vi "Accelerometer Logger.vi"() -> ()   [LabVIEW 2013]
uses:
  Accelerometer Data.ctl
  <vilib>/Platform/TimedLoop/XDataNode/timing_clust.ctl
  <vilib>/Platform/TimedLoop/XDataNode/nitl_modes.ctl
  <vilib>/Platform/TimedLoop/XDataNode/wakeup.ctl
  <vilib>/Analysis/_algsub.llb/Real Vector Norm.vi
  <vilib>/platform/TimedLoop/XDataNode/XDataNode.xnode
  <vilib>/Platform/TimedLoop/XDataNode/XDNodeRunTimeDep.lvlib
  <vilib>/Analysis/NI_AALPro.lvlib
panel:
  in  "ACK timeout":dbl[unit]=0.5
  in  "I2C clock speed":dbl[unit]=100000.0
  in  "reset":bool
  out "file":path caption="File name:"
  in  "increment file":bool
  in  "Stop on trigger":bool=TRUE
  out "error out":errorcluster
  in  "zero":bool
  out "actrate":dbl[unit] caption="Actual rate"
  in  "Post trigger":dbl[unit]=0.5
  out "Trigger":bool
  out "mag":dbl(slide) caption="Magnitude (g)" scale=0.0..2.0
  in  "Stop":bool
  in  "accel range (g)":u16(ring)=2 items=["2"=2, "4"=4, "8"=8, "16"=16]
  in  "gyro range (deg/sec)":u16(ring)=250 items=["250"=250, "500"=500, "1000"=1000, "2000"=2000]
  out "Gyro":waveform(dbl)[](graph)
  out "Accel":waveform(dbl)[](graph)
  in  "Sampling rate":dbl[unit]=200.0
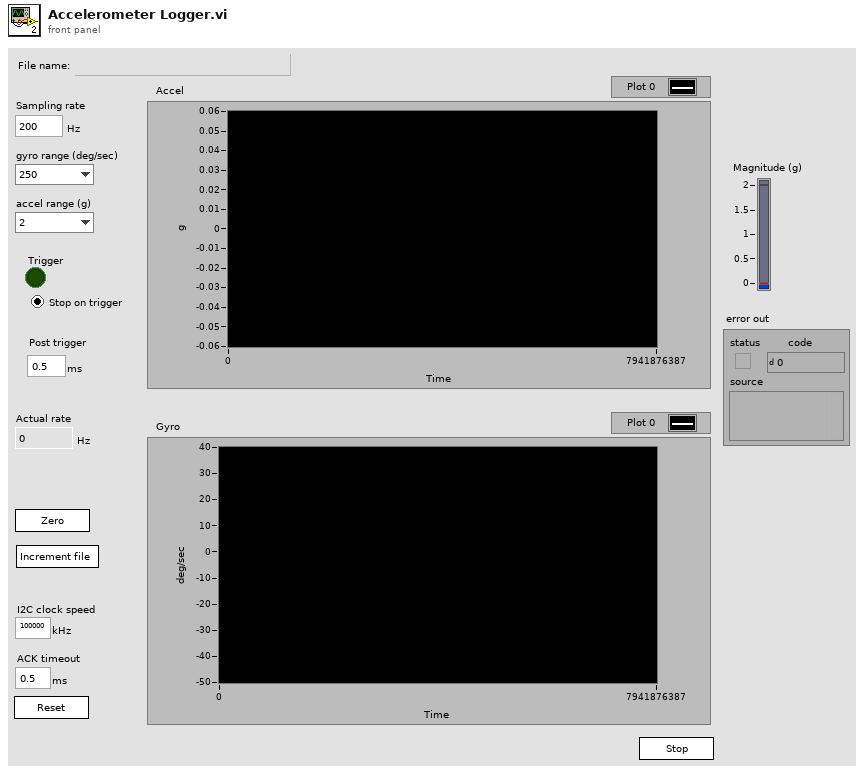
[diagram p1: front panel]
types:
  T1 = typedef "Accelerometer Data.ctl" = cluster{"Accel":dbl[], "Gyro":dbl[], "Time":u64, "Trigger":bool}
  T2 = typedef "Accelerometer.ctl" = cluster{"Device":T3, "i2c configuration":T4}
  T3 = typedef "ni845xControl.ctl" = refnum<k21>
  T4 = typedef "ni845xI2cConfiguration.ctl" = refnum<k20>
  T5 = typedef "XDNodeRunTimeDep.lvlib/timing_clust.ctl" = cluster{"Expected End [f-1]":u64, "Actual End [f-1]":u64, "Finished Late? [f-1]":bool, "Expected End [i-1]":u64, "Actual End [i-1]":u64, "Finished Late? [i-1]":bool, "Expected Start [i]":u64, "Actual Start [i]":u64, "Expected Start [f]":u64, "Actual Start [f]":u64, "Source Name":string, "Structure Name":string, "Period":i64, "Deadline":i64, "Offset":i64, "Start":i64, "Priority":i32, "Timeout":i32, "Mode":T6, "Wakeup Reason":T7, "Error":errorcluster, "Source Type":string, "Secondary Source Type":string, "Global End Time":u64, "Global Start Time":u64, "Frame Duration":u64, "Iteration Duration":u64, "Assigned CPU":i32, "I/O Scan Engine Mode":u32}
  T6 = typedef "XDNodeRunTimeDep.lvlib/nitl_modes.ctl" = enum32{"No Change", "Process missed periods, maintain original phase", "Discard missed periods, maintain original phase", "Process missed periods, ignore original phase", "Discard missed periods, ignore original phase"}
  T7 = typedef "XDNodeRunTimeDep.lvlib/wakeup.ctl" = enum32{"Normal", "Aborted", "Asynchronous wakeup", "Timing source error", "Timed loop error", "Timeout"}
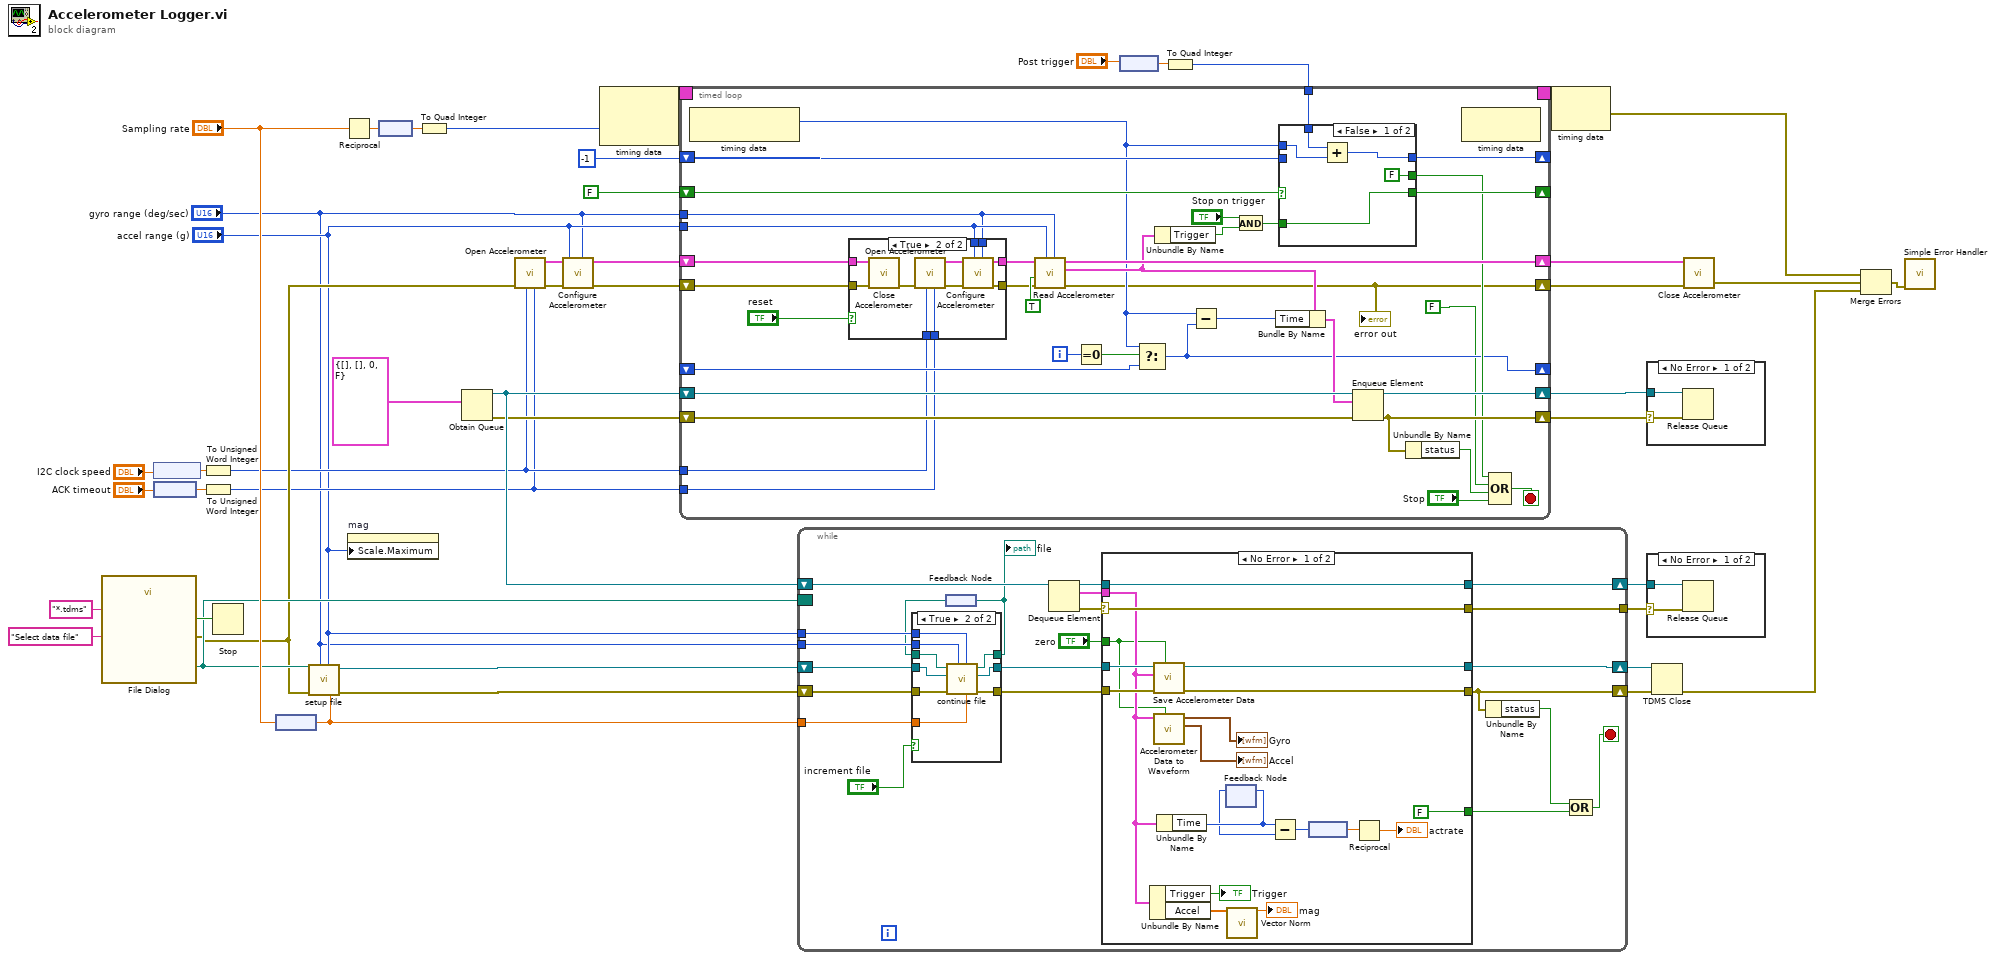
[diagram p0: block diagram]
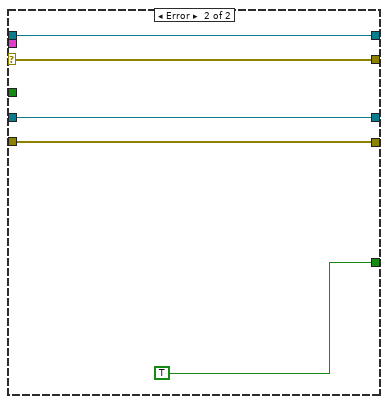
[diagram p5: hidden frame]
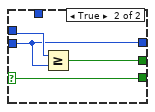
[diagram p7: hidden frame]
diagram:
  n1 = call "File Dialog"("prompt"="Select data file", "pattern (all files)"="*.tdms") -> ("selected path"=w14:path, "cancelled"=w34:bool, "error out"=w6:errorcluster)  [unwired: 10 in, 1 out]
  n2 = node("I2C clock speed") -> (w12:dbl)
  n3 = node("ACK timeout") -> (w13:dbl)
  n4 = To Unsigned Word Integer(number=w12) -> (unsigned 16bit integer=w5:u16)
  n5 = To Unsigned Word Integer(number=w13) -> (unsigned 16bit integer=w4:u16)
  n6 = Stop(stop? (T)=w34) -> ()
  n7 = node("Sampling rate") -> (w15:dbl)
  n8 = call "setup file.vi"("sampling rate"=w15, "accel range"="accel range (g)", "gyro range"="gyro range (deg/sec)", "error in (no error)"=w6, "selected path"=w14) -> ("error out"=w32:errorcluster, "tdms file out"=w33:refnum<k34>)  [unwired: 4 in, 1 out]
  n9 = Reciprocal(x="Sampling rate") -> (1/x=w44:dbl[unit])
  n10 = property on="mag" class="Slide (strict)"("Scale.Maximum"="accel range (g)") -> ()  [unwired: 2 in, 2 out]
  n11 = node(w44) -> (w43:dbl)
  n12 = To Quad Integer(1:w43) -> (0:w42:i64)
  n13 = Obtain Queue(element data type=T1 {"Accel"=[], "Gyro"=[], "Time"=0, "Trigger"=FALSE} ("Accelerometer Data")) -> (queue out=w40:refnum<queue>, error out=w39:errorcluster)  [unwired: 4 in, 1 out]
  n14 = call "Open Accelerometer.vi"("ACK Poll Timeout"=w4, "Clock Rate in kHz"=w5, "error in (no error)"=w6) -> ("error out"=w7:errorcluster, "Accelerometer"=w3:T2)  [unwired: 7 in]
  n15 = call "Configure Accelerometer.vi"("gyro range (deg/sec)"="gyro range (deg/sec)", "accel range (g)"="accel range (g)", "error in (no error)"=w7, "Accelerometer"=w3) -> ("error out"=w8:errorcluster, "Accelerometer out"=w9:T2)  [unwired: 6 in]
  n16 = node-c288(w42) -> (w46:T5)  [unwired: 1 in]
  n17 = while {
    shift-right: [w65] -> w28
    shift-left: w40 -> [w68]
    shift-right: [w50] -> w30
    shift-left: w33 -> [w58]
    shift-right: [w49] -> w31
    shift-left: w32 -> [w57]
    tunnel: [w60] -> w29
    tunnel: "gyro range (deg/sec)" -> [w54]
    tunnel: "accel range (g)" -> [w53]
    tunnel: w15 -> [w52]
    border: w14 -> [_]
    stop <- w63 stop-if-true
    n18 = feedback #1() -> (w48:path)
    n19 = case shown="True" "increment file" {
      tunnel: w58 -> [w71 w74]
      tunnel: w57 -> [w70 w80]
      tunnel: [w71 w72] -> w56
      tunnel: [w70 w79] -> w55
      tunnel: w54 -> [_ w78]
      tunnel: w53 -> [_ w77]
      tunnel: w52 -> [_ w76]
      tunnel: w48 -> [w69 w75]
      tunnel: [w69 w73] -> w47
      frame False {
      }
      frame True {
        n20 = call "continue file.vi"("sampling rate"=w76, "accel range"=w77, "gyro range"=w78, "error in (no error)"=w80, "original file"=w74, "original path"=w75) -> ("error out"=w79:errorcluster, "tdms file out"=w72:refnum<k34>, "incremented path"=w73:path)  [unwired: 2 in, 1 out]
      }
    }
    "file" <- w47
    n21 = feedback-in #1(w47) -> ()
    n22 = Dequeue Element(queue=w68) -> (queue out=w64:refnum<queue>, element=w66:T1, error out=w67:errorcluster)  [unwired: 2 in, 1 out]
    n23 = case shown="No Error" w67 {
      selector: w67 -> [w92 w100]
      tunnel: w66 -> [w87 _]
      tunnel: [FALSE TRUE] -> w62
      tunnel: w56 -> [w97 w102]
      tunnel: w55 -> [w96 w101]
      tunnel: [w95 w102] -> w50
      tunnel: [w94 w101] -> w49
      tunnel: [w93 w103] -> w65
      tunnel: w64 -> [w93 w103]
      tunnel: [w92 w100] -> w60
      tunnel: "zero" -> [w81 _]
      frame No Error {
        n24 = Unbundle By Name(w87) -> ("Trigger"=→"Trigger":bool, "Accel"=w91:dbl[])
        n25 = call "Save Accelerometer Data.vi"("zero"=w81, "error in (no error)"=w96, "Accelerometer Data"=w87, "tdms file"=w97) -> ("error out"=w94:errorcluster, "tdms file out"=w95:refnum<k34>)  [unwired: 6 in]
        n26 = call "Accelerometer Data to Waveform.vi"("zero"=w81, "Accelerometer Data"=w87) -> ("accel plot"=→"Accel":waveform(dbl)[], "gyro plot"=→"Gyro":waveform(dbl)[])  [unwired: 8 in]
        n27 = Unbundle By Name(w87) -> ("Time"=w86:u64)
        n28 = feedback-in #2(w86) -> ()
        n29 = feedback #2() -> (w85:u64)  [unwired: 1 in]
        n30 = call-poly <vilib>:"Vector Norm.vi"("Input Vector"=w91) -> ("norm"=→"mag":dbl)  [unwired: 9 in, 1 out]
        n31 = Subtract(x=w86, y=w85) -> (x-y=w84:u64)
        n32 = node(w84) -> (w83:dbl[unit])
        n33 = Reciprocal(x=w83) -> (1/x=→"actrate":dbl[unit])
      }
      frame Error {
      }
    }
    n34 = Unbundle By Name(w49) -> ("status"=w61:bool)
    n35 = Compound Arithmetic op=OR(w61, w62) -> (w63:bool)
  }
  n36 = node("Post trigger") -> (w18:dbl)
  n37 = To Quad Integer(1:w18) -> (0:w17:i64)
  n38 = timed-loop {
    timing: w46 -> [_]
    timing-out: [_] -> w45
    tunnel: "accel range (g)" -> [w114]
    tunnel: "gyro range (deg/sec)" -> [w113]
    shift-right: [w135] -> w26
    shift-left: w39 -> [w139]
    shift-right: [w119] -> w37
    shift-left: w8 -> [w112]
    shift-right: [w138] -> w27
    shift-left: w40 -> [w140]
    shift-right: [w141] -> w38
    shift-left: w9 -> [w111]
    shift-right: [w127] -> _
    shift-left: i64 -1 -> [w131]
    shift-right: [w129] -> _
    shift-left: FALSE -> [w132]
    tunnel: w17 -> [w128]
    shift-right: [w122] -> _
    shift-left: _ -> [w123]
    tunnel: w5 -> [w107]
    tunnel: w4 -> [w106]
    i -> [w124]
    stop <- w137 stop-if-true
    n39 = node-c288() -> (w121:i64)  [unwired: 1 in]
    n40 = case shown="True" "reset" {
      tunnel: w114 -> [_ w152]
      tunnel: w113 -> [_ w151]
      tunnel: w112 -> [w142 w150]
      tunnel: w111 -> [w143 w149]
      tunnel: [w143 w148] -> w110
      tunnel: [w142 w147] -> w109
      tunnel: w107 -> [_ w146]
      tunnel: w106 -> [_ w145]
      frame False {
      }
      frame True {
        n41 = call "Close Accelerometer.vi"("error in (no error)"=w150, "Accelerometer"=w149) -> ("error out"=w144:errorcluster)  [unwired: 9 in]
        n42 = call "Open Accelerometer.vi"("ACK Poll Timeout"=w145, "Clock Rate in kHz"=w146, "error in (no error)"=w144) -> ("error out"=w153:errorcluster, "Accelerometer"=w154:T2)  [unwired: 7 in]
        n43 = call "Configure Accelerometer.vi"("gyro range (deg/sec)"=w151, "accel range (g)"=w152, "error in (no error)"=w153, "Accelerometer"=w154) -> ("error out"=w147:errorcluster, "Accelerometer out"=w148:T2)  [unwired: 6 in]
      }
    }
    n44 = call "Read Accelerometer.vi"("gyro range (deg/sec)"=w113, "accel range (g)"=w114, "error in (no error)"=w109, "check ready"=TRUE, "Accelerometer"=w110) -> ("error out"=w119:errorcluster, "Accelerometer Data"=w130:T1, "Accelerometer out"=w141:T2)  [unwired: 3 in, 1 out]
    "error out" <- w119
    n45 = Equal To 0?(x=w124) -> (x = 0?=w108:bool)
    n46 = Select(t=w121, s=w108, f=w123) -> (s? t:f=w122:i64)
    n47 = Unbundle By Name(w130) -> ("Trigger"=w117:bool)
    n48 = Subtract(x=w121, y=w122) -> (x-y=w125:i64)
    n49 = And(x="Stop on trigger", y=w117) -> (x .and. y?=w115:bool)
    n50 = Bundle By Name(cluster=w130, "Time"=w125) -> (w133:T1)
    n51 = case shown="False" w132 {
      selector: w132 -> [_ w161]
      tunnel: w121 -> [w157 w163]
      tunnel: w131 -> [_ w160]
      tunnel: [FALSE w162] -> w126
      tunnel: w115 -> [w159 _]
      tunnel: [w159 w161] -> w129
      tunnel: w128 -> [w158 _]
      tunnel: [w156 w160] -> w127
      frame False {
        n52 = Add(x=w158, y=w157) -> (x+y=w156:i64)
      }
      frame True {
        n53 = Greater Or Equal?(x=w163, y=w160) -> (x >= y?=w162:bool)
      }
    }
    n54 = Enqueue Element(queue=w140, element=w133, error in (no error)=w139) -> (queue out=w138:refnum<queue>, error out=w135:errorcluster)  [unwired: 1 in, 1 out]
    n55 = Unbundle By Name(w135) -> ("status"=w134:bool)
    n56 = node-c288() -> ()  [unwired: 1 in, 1 out]
    n57 = Compound Arithmetic op=OR(w126, FALSE ("value"), w134, "Stop") -> (w137:bool)
  }
  n58 = node-c288(w45) -> (w22:errorcluster)
  n59 = case shown="No Error" w26 {
    selector: w26 -> [w167 _]
    tunnel: w27 -> [w168 _]
    frame No Error {
      n60 = Release Queue(queue=w168, error in (no error)=w167) -> ()  [unwired: 1 in, 3 out]
    }
    frame Error {
    }
  }
  n61 = case shown="No Error" w29 {
    selector: w29 -> [w169 _]
    tunnel: w28 -> [w170 _]
    frame No Error {
      n62 = Release Queue(queue=w170, error in (no error)=w169) -> ()  [unwired: 1 in, 3 out]
    }
    frame Error {
    }
  }
  n63 = TDMS Close(8:w31, 11:w30) -> (0:w23:errorcluster)  [unwired: 1 out]
  n64 = call "Close Accelerometer.vi"("error in (no error)"=w37, "Accelerometer"=w38) -> ("error out"=w24:errorcluster)  [unwired: 9 in]
  n65 = Merge Errors(w22, w24, w23) -> (w25:errorcluster)
  n66 = call <vilib>:"Simple Error Handler.vi"("error in (no error)"=w25) -> ()  [unwired: 4 in, 5 out]
